vi "Configure Orientation.vi"(6 "Change Default value? (F)":bool, 8 "error in (no error)":errorcluster, 10 "Orientation":u8(ring) items=["Level Orientation", "Upright Edge Orientation", "Upright Front Orientation"], 11 "Honeywell Compass HMC6343":refnum<class "Honeywell Compass HMC6343.lvclass">) -> (0 "error out":errorcluster, 3 "Honeywell Compass HMC6343 out":refnum<class "Honeywell Compass HMC6343.lvclass">)   [LabVIEW 2019, in "Honeywell Compass HMC6343.lvclass"]
doc: "The HMC6343 provides for three standard mouting orientations, with a flat horizontal orientation (Level) as the factory default. The others are Upright Edge(UE) and Upright Front(UF). If you want to change the default value, you should enable change default value? Or else the setting will revert to the default value when power on next time."
uses:
  Honeywell Compass HMC6343.lvclass
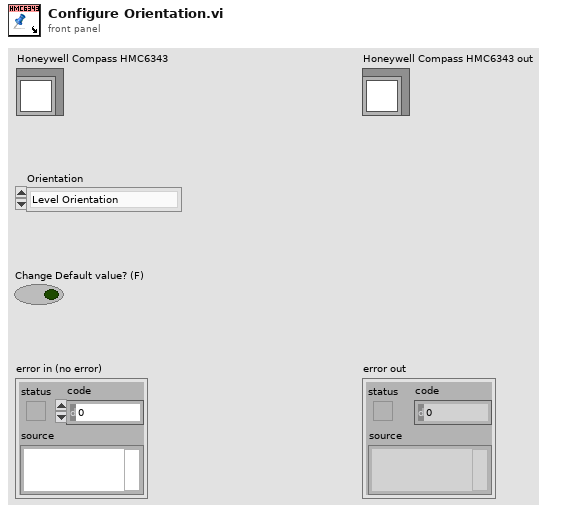
[diagram p1: front panel]
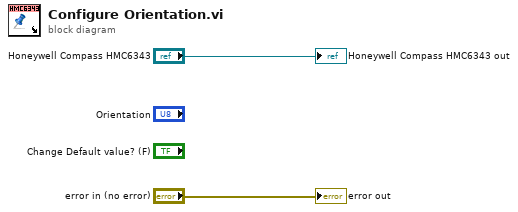
[diagram p0: block diagram]
diagram:
  "error out" <- "error in (no error)"
  "Honeywell Compass HMC6343 out" <- "Honeywell Compass HMC6343"
